vi "Parse Command.vi"(11 "text":string) -> (1 "Commands":string[](array[string]), 2 "flute dia (in)":dbl, 3 "cmd amd State":cluster{"Command":string, "End State":dbl[]}[](array[cluster]))   [LabVIEW 2024]
uses:
  <vilib>/Utility/error.llb/Trim Whitespace One-Sided.vi
panel:
  out "inch?":bool
  out "header":string[](array[string])
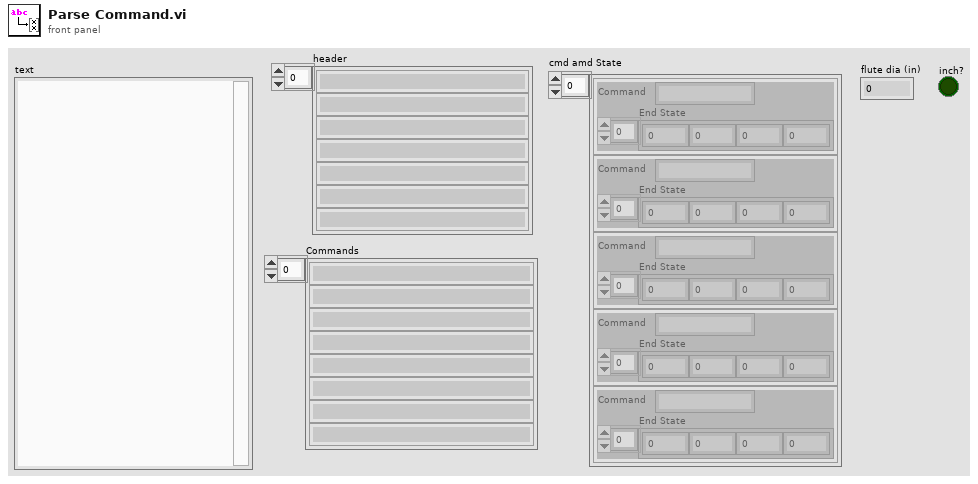
[diagram p1: front panel]
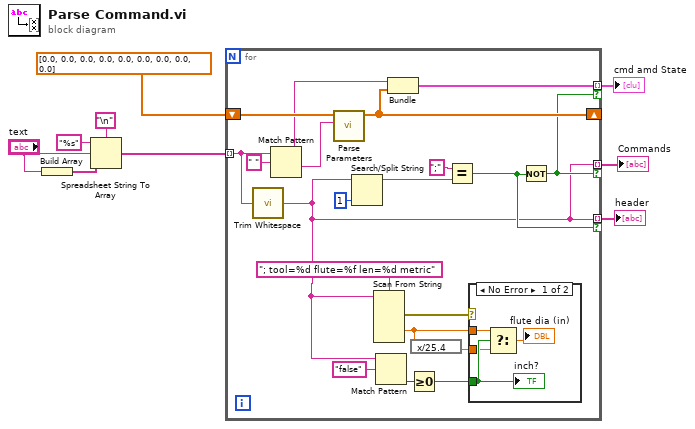
[diagram p0: block diagram]
diagram:
  n1 = Build Array("text") -> (w6:string[])
  n2 = Spreadsheet String To Array(delimiter (Tab)="\n", format string="%s", spreadsheet string="text", array type (2D Dbl)=w6) -> (array=w2:string[])
  n3 = for {
    tunnel: w2 -> [w23] mode=indexing
    shift-right: [w25] -> _
    shift-left: dbl[] [0.0, 0.0, 0.0, 0.0, 0.0, 0.0, 0.0, 0.0, 0.0] -> [w27]
    tunnel: [w24] -> w4 mode=indexing if=w13
    tunnel: [w10] -> w3 mode=indexing if=w20
    tunnel: [w10] -> w1 mode=indexing if=w13
    n4 = call <vilib>:"Trim Whitespace.vi"("string"=w23) -> ("trimmed string"=w10:string)  [unwired: 1 in]
    n5 = Match Pattern(string=w23, regular expression=" ") -> (before substring=w26:string, after substring=w28:string)  [unwired: 1 in, 2 out]
    n6 = call "Parse Parameters.vi"("String"=w28, "Array in"=w27) -> ("Array out"=w25:dbl[])  [unwired: 9 in]
    n7 = Search/Split String(string=w10, offset (0)=1) -> (substring before match=w12:string)  [unwired: 1 in, 2 out]
    n8 = Scan From String(format string="; tool=%d flute=%f len=%d metric" ("regular expression"), input string=w10) -> (error out=w18:errorcluster, output 2=w11:dbl)  [unwired: 7 in, 2 out]
    n9 = Match Pattern(string=w10, regular expression="false") -> (offset past match=w16:i32)  [unwired: 1 in, 3 out]
    n10 = Bundle("text"=w26, "Array out"=w25) -> (w24:cluster{"text":string, "Array out":dbl[]})  [unwired: 1 in]
    n11 = Greater Or Equal To 0?(x=w16) -> (x >= 0?=w15:bool)
    n12 = expression code="x/25.4"(w11) -> (w14:dbl)
    n13 = Equal?(x=";", y=w12) -> (x = y?=w20:bool)
    n14 = case shown="No Error" w18 {
      tunnel: w11 -> [w33 _]
      tunnel: w15 -> [w32 _]
      tunnel: w14 -> [w30 _]
      frame No Error {
        n15 = Select(t=w33, s=w32, f=w30) -> (s? t:f=→"flute dia (in)":dbl)
        "inch?" <- w32
      }
      frame Error {
      }
    }
    n16 = Not(x=w20) -> (.not. x?=w13:bool)
  }
  "Commands" <- w1
  "cmd amd State" <- w4
  "header" <- w3
